vi "TempMonitor_SetLimits_SetTemp_CheckSerialAlert.vi"(0 "Serial Port to Use":refnum<visa-resource-name>="COM8", 1 "High Limit (C)":i32=60, 2 "Low Limit (C)":i32=-10, 3 "Sensor Temp (C)":dbl, 4 "Test Block Analog Output":tag="Dev1/ao0") -> (14 "Pass":bool, 19 "error out":errorcluster)   [LabVIEW 2012]
uses:
  <vilib>/DAQmx/write.llb/DAQmx Write (Analog DBL 1Chan 1Samp).vi
  TempMonitor_Command_Enumerations.vi
  <vilib>/DAQmx/create/channels.llb/DAQmx Create Channel (AO-Voltage-Basic).vi
  <vilib>/DAQmx/miscellaneous.llb/DAQmx Fill In Error Info.vi
panel:
  out "Ack Received 2":bool
  out "Layer2 Payload 2":string
  out "A Packet Acked 2":bool
  out "Layer2 Payload 1":string
  out "Ack Received 1":bool
  out "A Packet Acked 1":bool
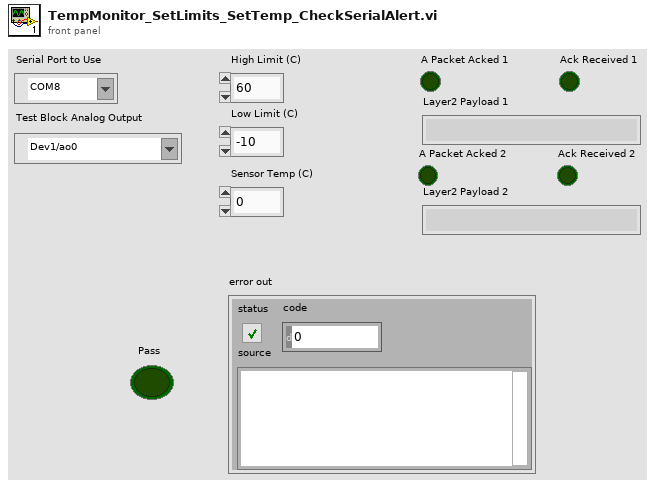
[diagram p1: front panel]
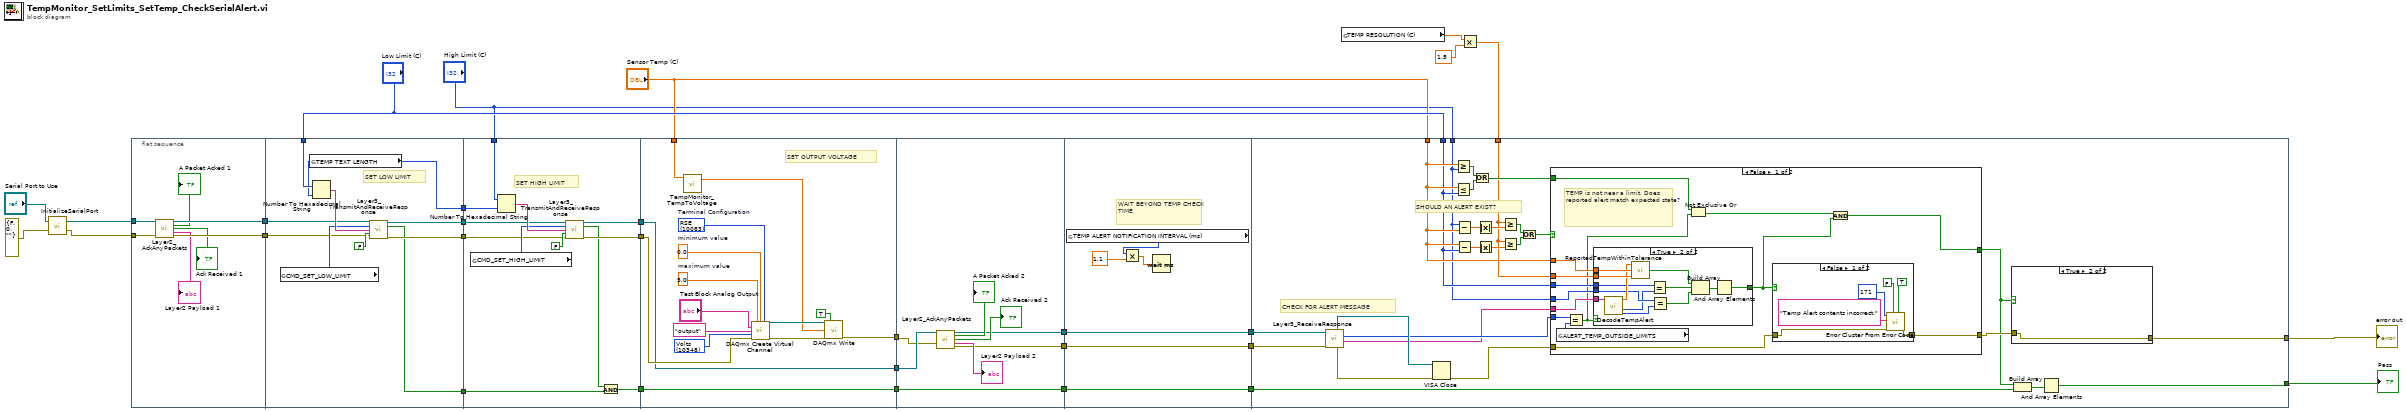
[diagram p0: block diagram]
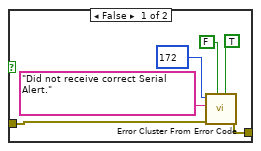
[diagram p2: hidden frame]
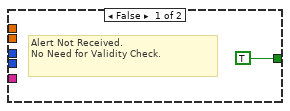
[diagram p4: hidden frame]
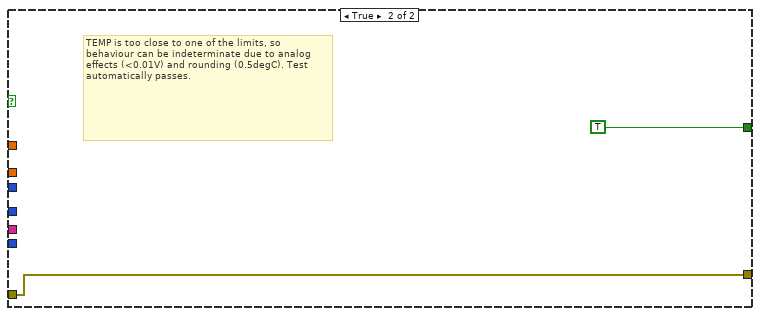
[diagram p5: hidden frame]
diagram:
  n1 = call "InitializeSerialPort.vi"("error in (no error)"=errorcluster {"status"=FALSE, "code"=0, "source"=""}, "Serial Port to Use"="Serial Port to Use") -> ("error out"=w23:errorcluster, "Configured Serial Port Identifier"=w22:refnum<visa-resource-name>)
  n2 = flat-sequence {
    tunnel: [w37] -> w25
    tunnel: [w36] -> w24
    tunnel: w23 -> [w35]
    tunnel: w22 -> [w34]
    tunnel: [w39] -> w14
    tunnel: "Low Limit (C)" -> [w44]
    tunnel: [w43] -> w12
    tunnel: [w42] -> w10
    tunnel: w25 -> [w41]
    tunnel: w24 -> [w40]
    tunnel: [w38] -> w7
    tunnel: w14 -> [w48]
    tunnel: [w50] -> w13
    tunnel: w12 -> [w56]
    tunnel: [w55] -> w11
    tunnel: w10 -> [w53]
    tunnel: [w54] -> w9
    tunnel: "High Limit (C)" -> [w52]
    tunnel: w7 -> [w51]
    tunnel: w13 -> [w61]
    tunnel: w11 -> [w60]
    tunnel: w9 -> [w63]
    tunnel: "Sensor Temp (C)" -> [w64]
    tunnel: [w62] -> w17
    tunnel: [w61] -> w16
    tunnel: [w60] -> w15
    tunnel: [w79] -> w6
    tunnel: [w77] -> w4
    tunnel: [w76] -> w2
    tunnel: w17 -> [w75]
    tunnel: w16 -> [w79]
    tunnel: w15 -> [w78]
    tunnel: w6 -> [w88]
    tunnel: [w88] -> w5
    tunnel: w4 -> [w87]
    tunnel: [w87] -> w3
    tunnel: w2 -> [w86]
    tunnel: [w86] -> w1
    tunnel: "Sensor Temp (C)" -> [w99]
    tunnel: "High Limit (C)" -> [w97]
    tunnel: "Low Limit (C)" -> [w98]
    tunnel: [w105] -> w28
    tunnel: [w102] -> w29
    tunnel: w19 -> [w100]
    tunnel: w5 -> [w104]
    tunnel: w3 -> [w94]
    tunnel: w1 -> [w95]
    frame #0 {
      n3 = call "Layer2_AckAnyPackets.vi"("Serial Port to Use"=w34, "Error In"=w35) -> ("Serial Port to Use (out)"=w37:refnum<visa-resource-name>, "A Packet Acked"=→"A Packet Acked 1":bool, "Ack Received"=→"Ack Received 1":bool, "Layer2 Payload"=→"Layer2 Payload 1":string, "Error Out"=w36:errorcluster)  [unwired: 9 in]
    }
    frame #1 {
      # "SET LOW LIMIT"
      n4 = global read "TempMonitor_Command_Enumerations.vi" "CMD_SET_LOW_LIMIT"() -> (w45:u16)
      n5 = global read "TempMonitor_Command_Enumerations.vi" "TEMP TEXT LENGTH"() -> (w38:u8)
      n6 = Number To Hexadecimal String(1:w38, 2:w44) -> (0:w46:string)
      n7 = call "Layer3_TransmitAndReceiveResponse.vi"("Serial Port to Use"=w41, "CMD"=w45, "Message"=w46, "Expecting Response"=FALSE, "error in (no error)"=w40) -> ("Serial Port to Use (out)"=w43:refnum<visa-resource-name>, "Success"=w39:bool, "Error Out"=w42:errorcluster)  [unwired: 6 in, 2 out]
    }
    frame #2 {
      # "SET HIGH LIMIT"
      n8 = global read "TempMonitor_Command_Enumerations.vi" "CMD_SET_HIGH_LIMIT"() -> (w57:u16)
      n9 = Number To Hexadecimal String(1:w51, 2:w52) -> (0:w58:string)
      n10 = call "Layer3_TransmitAndReceiveResponse.vi"("Serial Port to Use"=w56, "CMD"=w57, "Message"=w58, "Expecting Response"=FALSE, "error in (no error)"=w53) -> ("Serial Port to Use (out)"=w55:refnum<visa-resource-name>, "Success"=w49:bool, "Error Out"=w54:errorcluster)  [unwired: 6 in, 2 out]
      n11 = And(x=w49, y=w48) -> (x .and. y?=w50:bool)
    }
    frame #3 {
      w66 = 10083 items=["Default"=-1, "RSE"=10083, "Differential"=10106, "Pseudodifferential"=12529]  # Terminal Configuration
      w68 = 5.0  # maximum value
      w67 = 0.0  # minimum value
      w69 = 10348 items=["Volts"=10348, "From Custom Scale"=10065] ("units")
      # "SET OUTPUT VOLTAGE"
      n12 = call "TempMonitor_TempToVoltage.vi"("Temp (C)"=w64) -> ("Output Voltage"=w65:dbl)  [unwired: 3 in, 1 out]
      n13 = call-poly <vilib>:"DAQmx Create Virtual Channel.vi"("maximum value"=w68, "minimum value"=w67, "output terminal configuration"=w66, "physical channels"="Test Block Analog Output", "name to assign"="output", "units"=w69, "error in"=w63) -> ("task out"=w74:refnum<k21>, "error out"=w73:errorcluster)  [unwired: 7 in]
      n14 = call-poly <vilib>:"DAQmx Write.vi"("task/channels in"=w74, "auto start"=TRUE, "data"=w65, "error in"=w73) -> ("error out"=w62:errorcluster)  [unwired: 9 in, 2 out]
    }
    frame #4 {
      n15 = call "Layer2_AckAnyPackets.vi"("Serial Port to Use"=w78, "Error In"=w75) -> ("Serial Port to Use (out)"=w76:refnum<visa-resource-name>, "A Packet Acked"=→"A Packet Acked 2":bool, "Ack Received"=→"Ack Received 2":bool, "Layer2 Payload"=→"Layer2 Payload 2":string, "Error Out"=w77:errorcluster)  [unwired: 9 in]
    }
    frame #5 {
      # "WAIT BEYOND TEMP CHECK TIME"
      n16 = global read "TempMonitor_Command_Enumerations.vi" "TEMP ALERT NOTIFICATION INTERVAL (ms)"() -> (w85:u32)
      n17 = Multiply(x=w85, y=1.1) -> (x*y=w83:dbl)
      n18 = Wait (ms)(milliseconds to wait=w83) -> ()  [unwired: 1 out]
    }
    frame #6 {
      # "SHOULD AN ALERT EXIST?"
      # "CHECK FOR ALERT MESSAGE"
      n19 = call "Layer3_ReceiveResponse.vi"("Error In"=w94, "Serial Port to Use"=w95) -> ("Response Message"=w90:string, "Response CMD"=w91:u16, "Error Out"=w93:errorcluster, "Serial Port to Use (out)"=w92:refnum<visa-resource-name>)  [unwired: 5 in, 1 out]
      n20 = VISA Close(VISA resource name=w92, error in (no error)=w93) -> (error out=w101:errorcluster)
      n21 = Greater Or Equal?(x=w99, y=w97) -> (x >= y?=w115:bool)
      n22 = Less Or Equal?(x=w99, y=w98) -> (x <= y?=w114:bool)
      n23 = Subtract(x=w97, y=w99) -> (x-y=w113:dbl)
      n24 = Subtract(x=w99, y=w98) -> (x-y=w111:dbl)
      n25 = Or(x=w115, y=w114) -> (x .or. y?=w107:bool)
      n26 = Absolute Value(x=w113) -> (abs(x)=w112:dbl)
      n27 = Absolute Value(x=w111) -> (abs(x)=w110:dbl)
      n28 = Greater Or Equal?(x=w100, y=w112) -> (x >= y?=w108:bool)
      n29 = Greater Or Equal?(x=w100, y=w110) -> (x >= y?=w109:bool)
      n30 = Or(x=w108, y=w109) -> (x .or. y?=w106:bool)
      n31 = case shown="False" w106 {
        tunnel: w107 -> [w127 _]
        tunnel: [w123 TRUE] -> w89
        tunnel: w91 -> [w135 _]
        tunnel: w90 -> [w134 _]
        tunnel: w101 -> [w129 w158]
        tunnel: w100 -> [w133 _]
        tunnel: w99 -> [w132 _]
        tunnel: w98 -> [w131 _]
        tunnel: w97 -> [w130 _]
        tunnel: [w128 w158] -> w96
        frame False {
          # "TEMP is not near a limit. Does reported alert match expected state?"
          n32 = global read "TempMonitor_Command_Enumerations.vi" "ALERT_TEMP_OUTSIDE_LIMITS"() -> (w136:u16)
          n33 = Equal?(x=w135, y=w136) -> (x = y?=w126:bool)
          n34 = case shown="True" w126 {
            tunnel: w134 -> [_ w157]
            tunnel: w133 -> [_ w156]
            tunnel: w132 -> [_ w155]
            tunnel: w131 -> [_ w153]
            tunnel: w130 -> [_ w152]
            tunnel: [TRUE w145] -> w124
            frame False {
              # "Alert Not Received.\nNo Need for Validity Check."
            }
            frame True {
              n35 = call "DecodeTempAlert.vi"("Message"=w157) -> ("High Limit"=w150:i16, "Low Limit"=w151:i16, "Temperature"=w154:dbl)  [unwired: 8 in]
              n36 = call "ReportedTempWithinTolerance.vi"("Temp Tolerance (C)"=w156, "Set Temp (C)"=w155, "Reported Temp (C)"=w154) -> ("Pass"=w149:bool)
              n37 = Equal?(x=w153, y=w151) -> (x = y?=w148:bool)
              n38 = Equal?(x=w152, y=w150) -> (x = y?=w147:bool)
              n39 = Build Array(w149, w148, w147) -> (w146:bool[])
              n40 = And Array Elements(Boolean array=w146) -> (logical AND=w145:bool)
            }
          }
          n41 = Not Exclusive Or(1:w126, 2:w127) -> (0:w125:bool)
          n42 = case shown="False" w124 {
            tunnel: w129 -> [w137 w143]
            tunnel: [w140 w143] -> w128
            frame False {
              n43 = call <vilib>:"Error Cluster From Error Code.vi"("is warning? (False)"=TRUE, "show call chain? (False)"=FALSE, "error in (no error)"=w137, "error message (\"\")"="Temp Alert contents incorrect." ("source"), "error code (0)"=171 ("code")) -> ("error out"=w140:errorcluster)  [unwired: 4 in]
            }
            frame True {
            }
          }
          n44 = And(x=w125, y=w124) -> (x .and. y?=w123:bool)
        }
        frame True {
          # "TEMP is too close to one of the limits, so behaviour can be indeterminate due to analog effects (<0.01V) and rounding (0.5degC). Test automatically passes."
        }
      }
      n45 = case shown="True" w89 {
        tunnel: [w119 w122] -> w105
        tunnel: w96 -> [w116 w122]
        frame False {
          n46 = call <vilib>:"Error Cluster From Error Code.vi"("is warning? (False)"=TRUE, "show call chain? (False)"=FALSE, "error in (no error)"=w116, "error message (\"\")"="Did not receive correct Serial Alert." ("source"), "error code (0)"=172 ("code")) -> ("error out"=w119:errorcluster)  [unwired: 4 in]
        }
        frame True {
        }
      }
      n47 = Build Array(w89, w104) -> (w103:bool[])
      n48 = And Array Elements(Boolean array=w103) -> (logical AND=w102:bool)
    }
  }
  n49 = global read "TempMonitor_Command_Enumerations.vi" "TEMP RESOLUTION (C)"() -> (w21:dbl)
  n50 = Multiply(x=w21, y=1.5) -> (x*y=w19:dbl)
  "Pass" <- w29
  "error out" <- w28
